vi "Write configuration.vi"(8 "error in":errorcluster, 10 "configuration":refnum<class "NISE_CEF_serializable configuration.lvclass">, 11 "PLTarget cDAQ in":refnum<class "PLTarget PXI.lvclass">) -> (0 "error out":errorcluster, 3 "PLTarget cDAQ out":refnum<class "PLTarget PXI.lvclass">)   [LabVIEW 2013, in "PLTarget PXI.lvclass"]
uses:
  PLTarget PXI.lvclass
  <vilib>/NI/Configuration Framework/serializable configuration/NISE_CEF_serializable configuration.lvclass
  Framework Configuration Classes/target configuration/PL_Target Configuration.lvclass
  PLTarget PXI.lvclass/PLTarget PXI.ctl
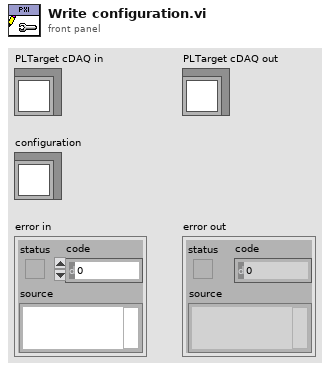
[diagram p1: front panel]
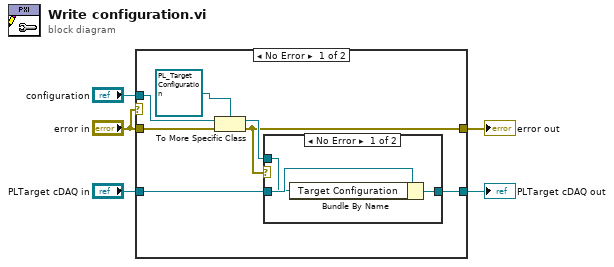
[diagram p0: block diagram]
diagram:
  n1 = case shown="No Error" "error in" {
    tunnel: "PLTarget cDAQ in" -> [w11 w18]
    tunnel: [w10 w18] -> w4
    tunnel: "configuration" -> [w9 _]
    tunnel: "error in" -> [w7 w17]
    tunnel: [w6 w17] -> w2
    frame No Error {
      n2 = To More Specific Class(target class=refnum<class "PL_Target Configuration.lvclass"> refnum ("Target Configuration"), reference=w9, error in=w7) -> (specific class reference=w8:refnum<class "PL_Target Configuration.lvclass">, error out=w6:errorcluster)
      n3 = case shown="No Error" w6 {
        tunnel: w11 -> [w15 w16]
        tunnel: [w14 w16] -> w10
        tunnel: w8 -> [w13 _]
        frame No Error {
          n4 = Bundle By Name(cluster=w15, "Target Configuration"=w13) -> (w14:refnum<class "PLTarget PXI.lvclass">)
        }
        frame Error {
        }
      }
    }
    frame Error {
    }
  }
  "error out" <- w2
  "PLTarget cDAQ out" <- w4
